vi "译码显示电路基本逻辑功能验证.vi"() -> ()   [LabVIEW 2018]
panel:
  in  "结束":bool
  in  "D":bool
  in  "C":bool
  in  "B":bool
  in  "A":bool
  out "c":bool
  out "e":bool
  out "d":bool
  out "g":bool
  out "b":bool
  out "f":bool
  out "a":bool
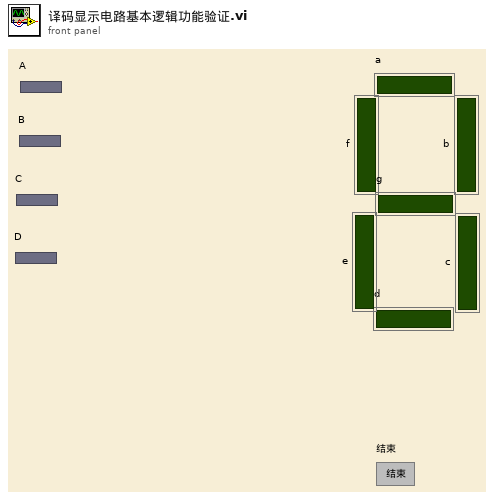
[diagram p1: front panel]
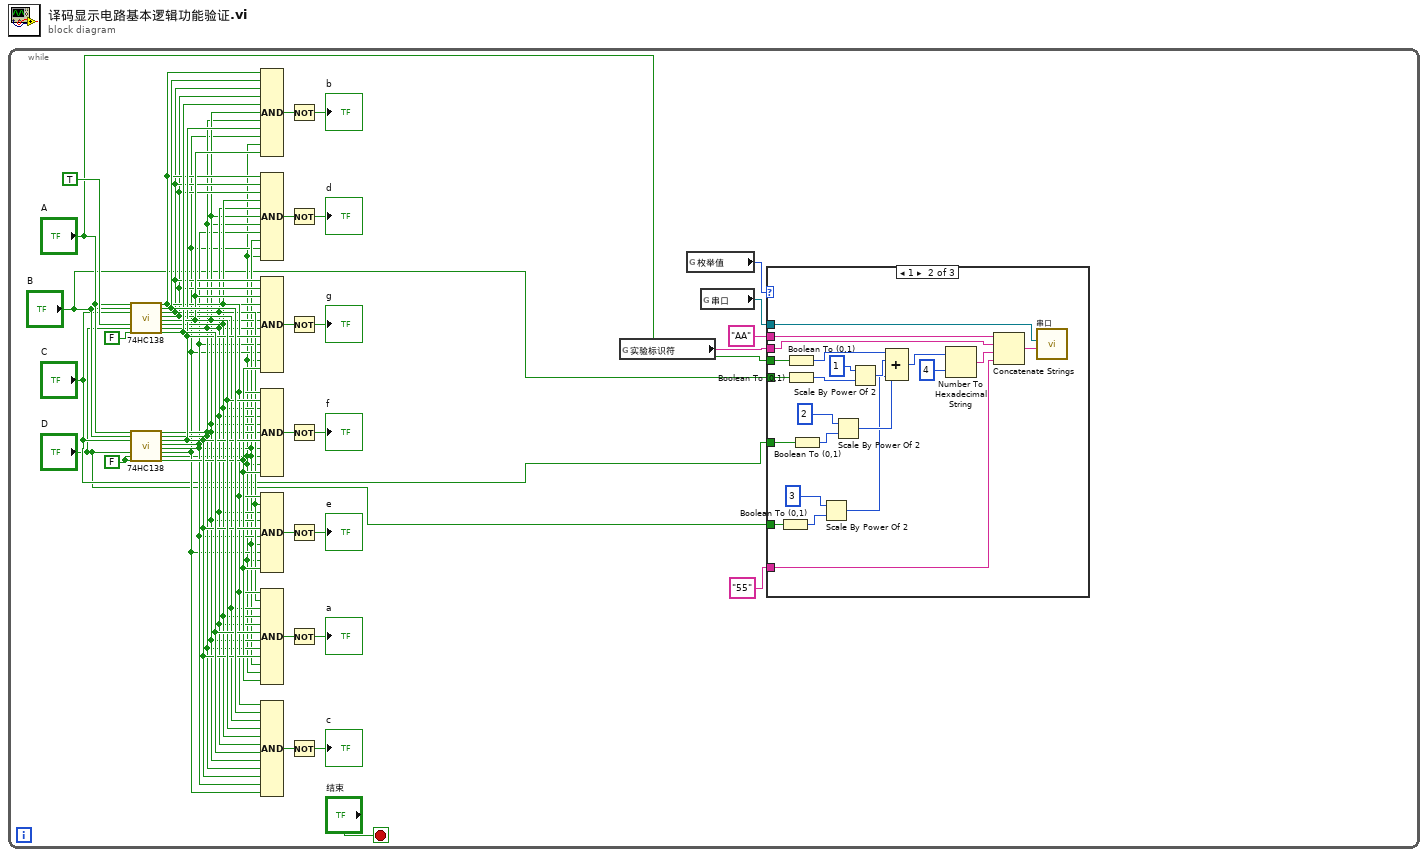
[diagram p0: block diagram]
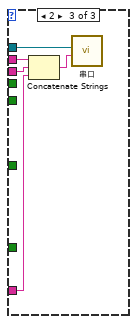
[diagram p3: hidden frame]
diagram:
  n1 = while {
    stop <- "结束" stop-if-true
    w41 = FALSE
    n2 = call "74HC138.vi"("A0"="A", "A1"="B", "A2"="C", "S1"=TRUE, "S2`"="D", "S3`"=FALSE) -> ("Y0`"=w21:bool, "Y1`"=w28:bool, "Y2`"=w20:bool, "Y3`"=w19:bool, "Y4`"=w24:bool, "Y5`"=w18:bool, "Y6`"=w17:bool, "Y7`"=w27:bool)  [unwired: 14 in]
    n3 = call "74HC138.vi"("A0"="A", "A1"="B", "A2"="C", "S1"="D", "S2`"=w41, "S3`"=w41) -> ("Y0`"=w16:bool, "Y1`"=w15:bool, "Y2`"=w23:bool, "Y3`"=w14:bool, "Y4`"=w13:bool, "Y5`"=w12:bool, "Y6`"=w11:bool, "Y7`"=w22:bool)  [unwired: 14 in]
    n4 = Compound Arithmetic op=AND ("复合运算")(w21, w28, w20, w19, w27, w16, w15, w23, w12, w11, w24) -> (w40:bool)
    n5 = Compound Arithmetic op=AND ("复合运算")(w21, w20, w19, w18, w17, w16, w15, w14, w13, w12, w11) -> (w34:bool)
    n6 = Compound Arithmetic op=AND ("复合运算")(w20, w19, w24, w18, w17, w16, w15, w23, w14, w12, w11, w22) -> (w33:bool)
    n7 = Compound Arithmetic op=AND ("复合运算")(w21, w24, w18, w17, w16, w15, w23, w14, w13, w11, w22) -> (w32:bool)
    n8 = Compound Arithmetic op=AND ("复合运算")(w21, w20, w17, w16, w23, w14, w13, w12, w11, w22) -> (w35:bool)
    n9 = Compound Arithmetic op=AND ("复合运算")(w21, w20, w19, w18, w17, w27, w16, w15, w23, w13, w11, w22) -> (w38:bool)
    n10 = Compound Arithmetic op=AND ("复合运算")(w21, w28, w19, w24, w18, w17, w27, w16, w15, w23, w14, w12) -> (w36:bool)
    n11 = Not(x=w40) -> (.not. x?=→"b":bool)
    n12 = Not(x=w34) -> (.not. x?=→"d":bool)
    n13 = Not(x=w33) -> (.not. x?=→"g":bool)
    n14 = Not(x=w32) -> (.not. x?=→"f":bool)
    n15 = Not(x=w35) -> (.not. x?=→"e":bool)
    n16 = Not(x=w38) -> (.not. x?=→"a":bool)
    n17 = Not(x=w36) -> (.not. x?=→"c":bool)
    n18 = global read "全局变量.vi" "实验标识符"() -> (w7:string)
    n19 = global read "全局变量.vi" "枚举值"() -> (w9:i8)
    n20 = global read "全局变量.vi" "串口"() -> (w8:refnum<visa-resource-name>)
    n21 = case shown="1" w9 {
      tunnel: "B" -> [_ w60 _]
      tunnel: "A" -> [_ w59 _]
      tunnel: w8 -> [_ w58 w68]
      tunnel: w7 -> [_ w57 w69]
      tunnel: "55" -> [_ w56 w66]
      tunnel: "AA" -> [_ w55 w67]
      tunnel: "C" -> [_ w49 _]
      tunnel: "D" -> [_ w44 _]
      frame 0, Default {
      }
      frame 1 {
        n22 = Boolean To (0,1)(Boolean=w44) -> (0, 1=w47:i16)
        n23 = Boolean To (0,1)(Boolean=w59) -> (0, 1=w64:i16)
        n24 = Boolean To (0,1)(Boolean=w60) -> (0, 1=w62:i16)
        n25 = Boolean To (0,1)(Boolean=w49) -> (0, 1=w50:i16)
        n26 = Scale By Power Of 2(n=3, x=w47) -> (x*2^n=w45:i16)
        n27 = Scale By Power Of 2(n=2, x=w50) -> (x*2^n=w51:i16)
        n28 = Scale By Power Of 2(n=1, x=w62) -> (x*2^n=w63:i16)
        n29 = Compound Arithmetic op=ADD ("复合运算")(w64, w63, w51, w45) -> (w54:i16)
        n30 = Number To Hexadecimal String(1:4, 2:w54) -> (0:w52:string)
        n31 = Concatenate Strings(w55, w57, w52, w56) -> (w65:string)
        n32 = call "串口.vi"("字符串"=w65, "VISA resource name"=w58) -> ()  [unwired: 10 in]
      }
      frame 2 {
        n33 = Concatenate Strings(w67, w69, w66) -> (w70:string)
        n34 = call "串口.vi"("字符串"=w70, "VISA resource name"=w68) -> ()  [unwired: 10 in]
      }
    }
  }
